vi "Write Picture.vi"(8 "error in (no error)":errorcluster, 10 "Picture":refnum<vi>, 11 "Image Gallery.lvclass in":refnum<class "Image Gallery.lvclass">) -> (0 "error out":errorcluster, 3 "Image Gallery.lvclass out":refnum<class "Image Gallery.lvclass">)   [LabVIEW 2012, in "ImageGallery.lvlib" / "Image Gallery.lvclass"]
uses:
  Image Gallery.lvclass
  Image Gallery.lvclass/Image Gallery.ctl
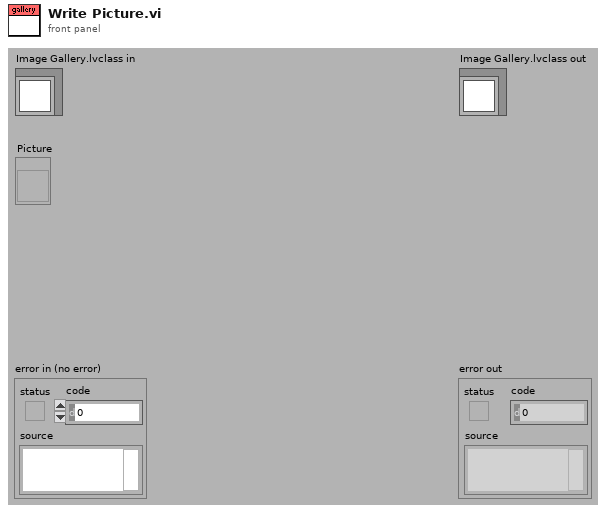
[diagram p1: front panel]
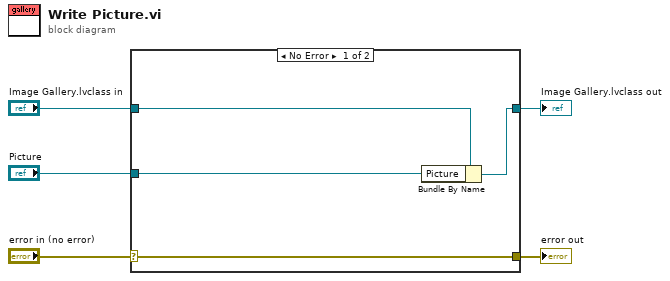
[diagram p0: block diagram]
diagram:
  n1 = case shown="No Error" "error in (no error)" {
    selector: "error in (no error)" -> [w9 w10]
    tunnel: [w9 w10] -> w4
    tunnel: [w7 w11] -> w2
    tunnel: "Image Gallery.lvclass in" -> [w8 w11]
    tunnel: "Picture" -> [w6 _]
    frame No Error {
      n2 = Bundle By Name(cluster=w8, "Picture"=w6) -> (w7:refnum<class "Image Gallery.lvclass">)
    }
    frame Error {
    }
  }
  "error out" <- w4
  "Image Gallery.lvclass out" <- w2
